vi "Copy Value.vi"(10 "From":refnum<class "Type.lvclass">, 11 "Entity Collection in":refnum<class "Entity Collection.lvclass">) -> (2 "error out":errorcluster, 3 "Entity Collection out":refnum<class "Entity Collection.lvclass">)   [LabVIEW 2020, in "Conditu2.lvlib" / "Columns.lvlib" / "Entity Collection.lvclass"]
uses:
  Entity Collection.lvclass
  Type/Type.lvclass
  Entity Collection.lvclass/Entity Collection.ctl
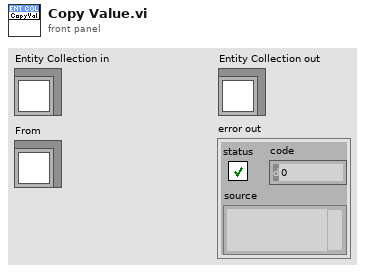
[diagram p1: front panel]
types:
  T1 = typedef "Conditu2.lvlib/Entity ID.ctl" = i64
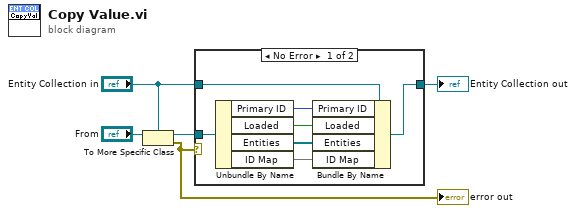
[diagram p0: block diagram]
diagram:
  n1 = To More Specific Class(target class="Entity Collection in", reference="From") -> (specific class reference=w4:refnum<class "Entity Collection.lvclass">, error out=w3:errorcluster)  [unwired: 1 in]
  "error out" <- w3
  n2 = case shown="No Error" w3 {
    tunnel: w4 -> [w12 _]
    tunnel: "Entity Collection in" -> [w11 w13]
    tunnel: [w6 w13] -> w1
    frame No Error {
      n3 = Unbundle By Name(w12) -> ("Primary ID"=w10:T1, "Loaded"=w9:bool, "Entities"=w8:refnum<class "Entity.lvclass">[], "ID Map"=w7:map{T1, i32})
      n4 = Bundle By Name(cluster=w11, "Primary ID"=w10, "Loaded"=w9, "Entities"=w8, "ID Map"=w7) -> (w6:refnum<class "Entity Collection.lvclass">)
    }
    frame Error {
    }
  }
  "Entity Collection out" <- w1
